vi "All Errors Read (library variable).vi"() -> ()   [LabVIEW 2023, in "Error Manager.lvlib"]
uses:
  Error Manager.lvlib
panel:
  out "All Errors Read?":bool
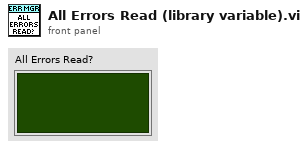
[diagram p1: front panel]
diagram:
